vi "Save.vi"(8 "error in (no error)":errorcluster, 9 "new command":string, 10 "Msg in":T1, 11 "FakeCamera in":refnum<class "MoveDataFile.lvclass">) -> (0 "error out":errorcluster, 1 "Path":path, 2 "Msg out":T1, 3 "FakeCamera out":refnum<class "MoveDataFile.lvclass">, 4 "new command":string)   [LabVIEW 2011, in "MoveDataFile.lvclass"]
uses:
  MoveDataFile.lvclass
  BaseDriver/DriverMsg.ctl
  MoveDataFile.lvclass/MoveDataFile.ctl
  BaseDriver/BaseDriver.lvclass
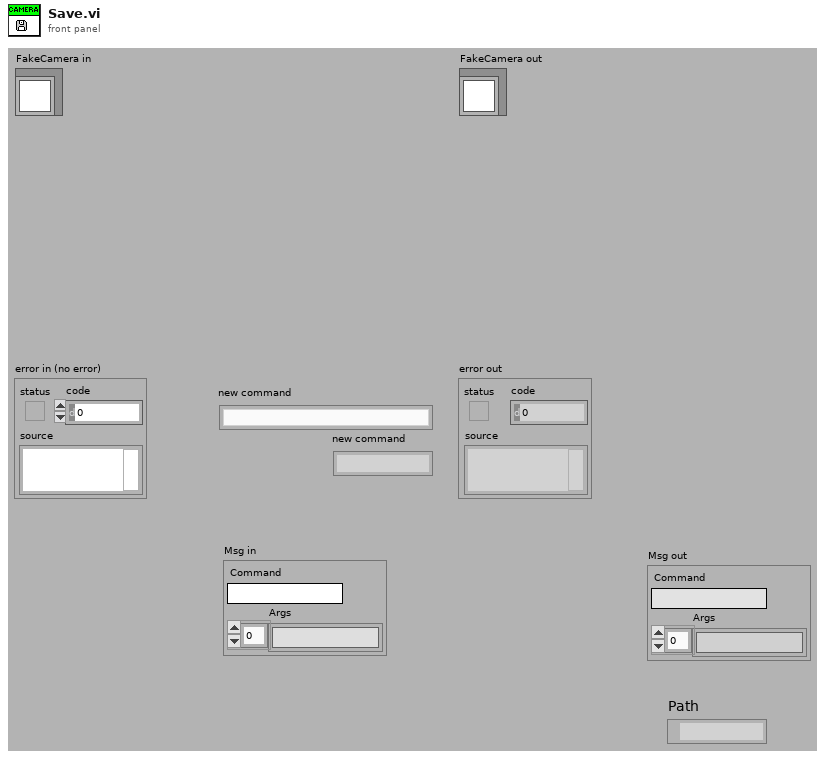
[diagram p1: front panel]
types:
  T1 = typedef "DriverMsg.ctl" = cluster{"Command":string, "Args":string[]}
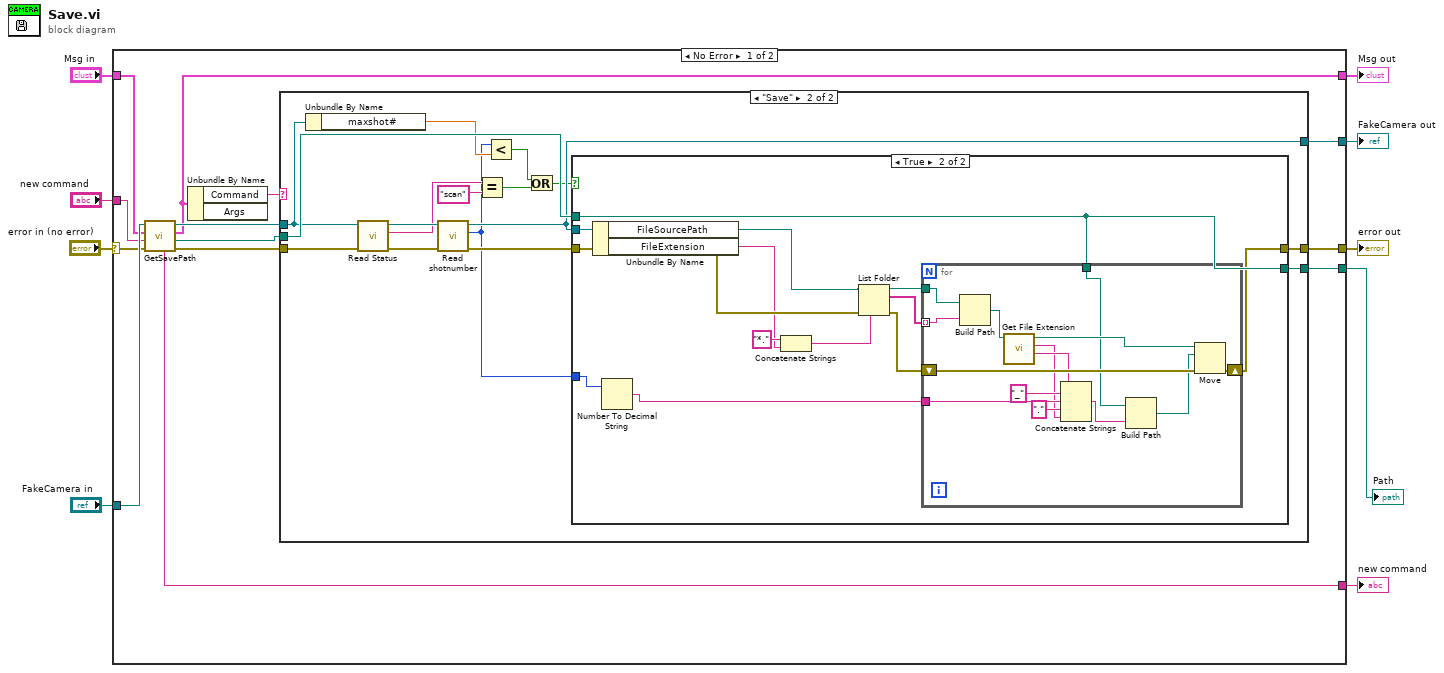
[diagram p0: block diagram]
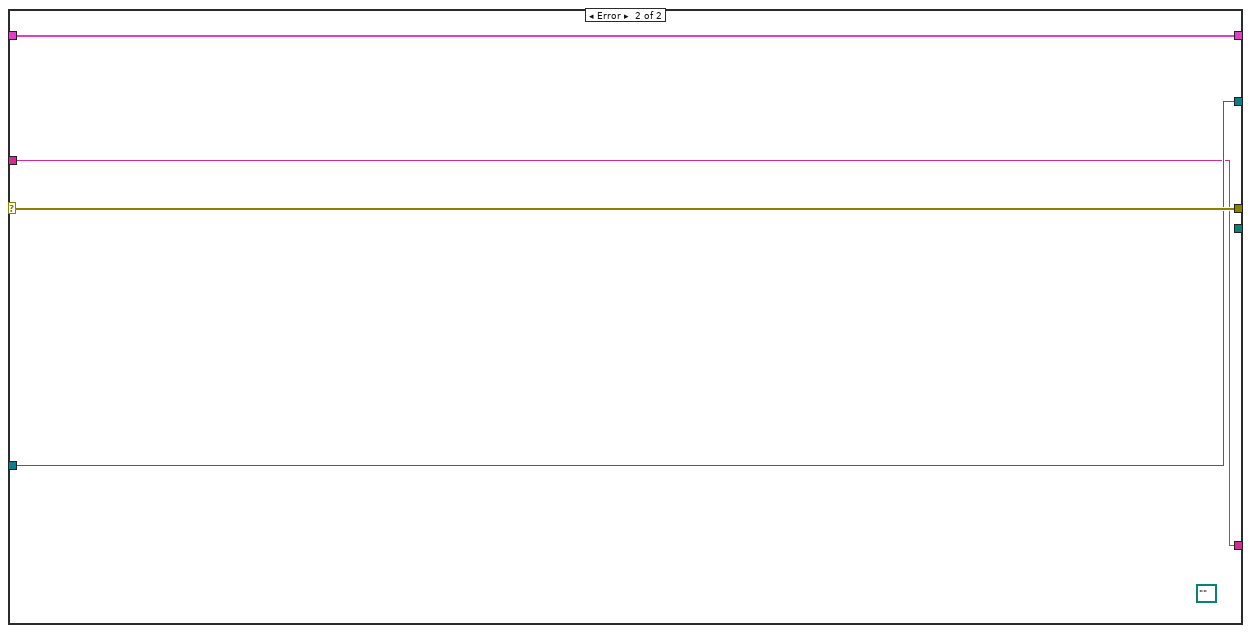
[diagram p4: hidden frame]
diagram:
  n1 = case shown="No Error" "error in (no error)" {
    selector: "error in (no error)" -> [w16 w72]
    tunnel: [w20 w72] -> w9
    tunnel: [w14 w71] -> w8
    tunnel: [w21 w70] -> w7
    tunnel: "Msg in" -> [w18 w71]
    tunnel: "FakeCamera in" -> [w19 w70]
    tunnel: "new command" -> [w17 w69]
    tunnel: [w11 w69] -> w2
    tunnel: [w10 _] -> w1
    frame No Error {
      n2 = call-dynamic "GetSavePath.vi"("error in (no error)"=w16, "new command"=w17, "Msg in"=w18, "BaseDriver in"=w19) -> ("error out"=w12:errorcluster, "Path"=w13:path, "Msg out"=w14:T1, "BaseDriver out"=w15:refnum<class "MoveDataFile.lvclass">, "new command"=w11:string)  [unwired: 3 in]
      n3 = Unbundle By Name(w14) -> ("Command"=w22:string)  [unwired: 1 out]
      n4 = case shown="\"Save\"" w22 {
        tunnel: w15 -> [w24 w36]
        tunnel: [w24 w38] -> w21
        tunnel: w13 -> [_ w40]
        tunnel: w12 -> [w23 w34]
        tunnel: [w23 w39] -> w20
        tunnel: [_ w26] -> w10
        frame Default {
        }
        frame "Save" {
          n5 = Unbundle By Name(w36) -> ("maxshot#"=w37:dbl)
          n6 = call "Read Status.vi"("error in (no error)"=w34, "BaseDriver in"=w36) -> ("error out"=w33:errorcluster, "Status"=w31:string, "BaseDriver out"=w35:refnum<class "MoveDataFile.lvclass">)  [unwired: 7 in]
          n7 = call-dynamic "Read shotnumber.vi"("error in (no error)"=w33, "BaseDriver in"=w35) -> ("error out"=w32:errorcluster, "shotnumber"=w25:i32, "BaseDriver out"=w38:refnum<class "MoveDataFile.lvclass">)  [unwired: 6 in, 1 out]
          n8 = Equal?(x=w31, y="scan" ("Status")) -> (x = y?=w29:bool)
          n9 = Less?(x=w25, y=w37) -> (x < y?=w28:bool)
          n10 = Or(x=w28, y=w29) -> (x .or. y?=w27:bool)
          n11 = case shown="True" w27 {
            tunnel: w40 -> [_ w45]
            tunnel: w32 -> [w41 w51]
            tunnel: [w41 w43] -> w39
            tunnel: w38 -> [_ w54]
            tunnel: [_ w45] -> w26
            tunnel: w25 -> [_ w53]
            frame False {
            }
            frame True {
              n12 = Unbundle By Name(w54) -> ("FileSourcePath"=w52:path, "FileExtension"=w49:string)
              n13 = Number To Decimal String(number=w53) -> (decimal integer string=w42:string)  [unwired: 1 in]
              n14 = Concatenate Strings("*." ("string"), w49) -> (w48:string)
              n15 = List Folder(path=w52, pattern=w48, error in=w51) -> (path out=w46:path, filenames=w47:string[], error out=w44:errorcluster)  [unwired: 1 in, 1 out]
              n16 = for {
                tunnel: w47 -> [w67] mode=indexing
                tunnel: w46 -> [w68]
                tunnel: w45 -> [w56]
                shift-right: [w65] -> w43
                shift-left: w44 -> [w66]
                tunnel: w42 -> [w63]
                n17 = Build Path(base path=w68, name or relative path=w67) -> (appended path=w58:path)
                n18 = call <vilib>:"Get File Extension.vi"("file"=w58) -> ("filename without extension"=w61:string, "lowercase file extension"=w59:string, "dup file"=w64:path)  [unwired: 7 in, 1 out]
                n19 = Concatenate Strings(w61, "_" ("string"), w63, "." ("string"), w59) -> (w57:string)
                n20 = Build Path(base path=w56, name or relative path=w57) -> (appended path=w55:path)
                n21 = Move(source path=w64, error in=w66, 10:w55) -> (error out=w65:errorcluster)  [unwired: 2 in, 2 out]
              }
            }
          }
        }
      }
    }
    frame Error {
      (unwired) path "" ("Path")
    }
  }
  "error out" <- w9
  "FakeCamera out" <- w7
  "Msg out" <- w8
  "new command" <- w2
  "Path" <- w1
